vi "Actor Receive Core.vi"(7 "Msg in":refnum<class "Msg Strategy.lvclass">, 11 "Destroying Self Actor State in":refnum<class "Destroying Self Actor State.lvclass">) -> (5 "Msg out":refnum<class "Msg Strategy.lvclass">)   [LabVIEW 2021, in "jettl.lvlib" / "Destroying Self Actor State.lvclass"]
uses:
  Destroying Self Actor State.lvclass
  Msg Strategy/Msg Strategy.lvclass
  Msgs/Actor Last Ack/Actor Last Ack Msg Strategy/Actor Last Ack Msg Strategy.lvclass
  C:/git/jettl/src_error_internal/LVCAM/LVCAM/Msg Strategy/Msg Strategy.lvclass
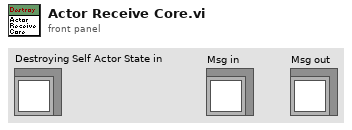
[diagram p1: front panel]
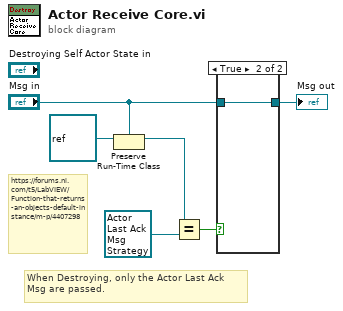
[diagram p0: block diagram]
diagram:
  # "https://forums.ni.com/t5/LabVIEW/Function-that-returns-an-objects-default-instance/m-p/4407298"
  # "When Destroying, only the Actor Last Ack Msg are passed."
  n1 = Preserve Run-Time Class(object in=refnum<class> refnum ("LabVIEW Object"), 2:"Msg in") -> (object out=w1:refnum<class "Msg Strategy.lvclass">)  [unwired: 1 in, 1 out]
  n2 = Equal?(x=w1, y=refnum<class "Actor Last Ack Msg Strategy.lvclass"> refnum ("LVCAM Nest Destroyed.lvlib:LVCAM Nest Destroyed Msg.lvclass")) -> (x = y?=w5:bool)
  n3 = case shown="True" w5 {
    tunnel: [_ w7] -> w6
    tunnel: "Msg in" -> [_ w7]
    frame False {
    }
    frame True {
    }
  }
  "Msg out" <- w6
